vi "_Raise Permission Requested.vi"(4 "WebView2.lvlib:WebView2 Control.lvclass":refnum<class "WebView2 Control.lvclass">, 5 "Event Data":cluster{"sender":refnum<k24>, "e":refnum<k24>}, 6 "Control Ref":refnum<k24>, 7 "Event Common Data":T1) -> ()   [LabVIEW 2025, in "WebView2.lvlib" / "WebView2 Control.lvclass"]
uses:
  WebView2 Control.lvclass
  WebView2 Control.lvclass/WebView2 Control.ctl
  E:/Labview/LV 2023/PPL/PPL Builder/Libs/LV-WebView2/Source/Libs/Microsoft.Web.WebView2.Core.dll
  Libs/Microsoft.Web.WebView2.Core.dll
  Permission Requested Event Data.ctl
  WebView2 Event Filter Interface/WebView2 Event Filter Interface.lvclass
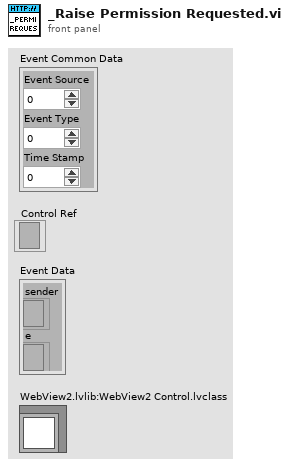
[diagram p1: front panel]
types:
  T1 = cluster{"Event Source":i32, "Event Type":u32, "Time Stamp":u32}
  T2 = typedef "WebView2.lvlib/WebView2 Control.lvclass/Permission Requested Event Data.ctl" = cluster{"IsUserInitiated":bool, "PermissionKind":i32, "Uri":string}
  T3 = cluster{"Handled":bool, "SavesInProfile":bool, "State":i32}
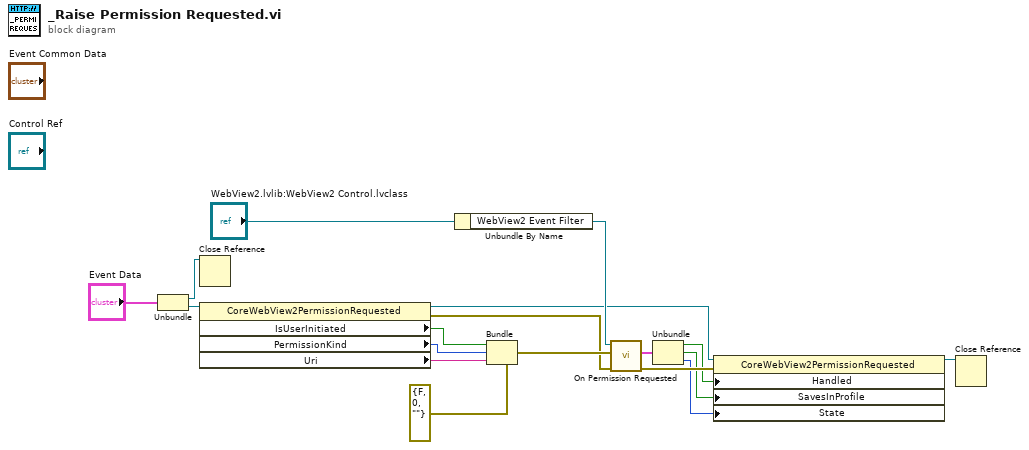
[diagram p0: block diagram]
diagram:
  n1 = Unbundle("Event Data") -> ("sender"=w17:refnum<k24>, "e"=w16:refnum<k24>)
  n2 = Close Reference(reference=w17) -> ()  [unwired: 1 in, 1 out]
  n3 = property class="CoreWebView2PermissionRequested"(reference=w16) -> (reference out=w7:refnum<k24>, error out=w10:errorcluster, "IsUserInitiated"=w15:bool, "PermissionKind"=w14:i32, "Uri"=w13:string)  [unwired: 1 in]
  n4 = Unbundle By Name("WebView2.lvlib:WebView2 Control.lvclass") -> ("WebView2 Event Filter"=w8:refnum<class "WebView2 Event Filter Interface.lvclass">)
  n5 = Bundle(cluster=T2 {"IsUserInitiated"=FALSE, "PermissionKind"=0, "Uri"=""}, "IsUserInitiated"=w15, "PermissionKind"=w14, "Uri"=w13) -> (w11:T2)
  n6 = call-dynamic "On Permission Requested.vi"("error in (no error)"=w10, "Data"=w11, "WebView2 Event Filter Interface in"=w8) -> ("error out"=w5:errorcluster, "Response"=w6:T3)  [unwired: 7 in]
  n7 = Unbundle(w6) -> ("Handled"=w4:bool, "SavesInProfile"=w3:bool, "State"=w2:i32)
  n8 = property class="CoreWebView2PermissionRequested"(reference=w7, error in=w5, "Handled"=w4, "SavesInProfile"=w3, "State"=w2) -> (reference out=w1:refnum<k24>)  [unwired: 1 out]
  n9 = Close Reference(reference=w1) -> ()  [unwired: 1 in, 1 out]
